vi "Idle_Password.vi"(2 "Called?":bool=TRUE) -> (0 "Correct?":bool, 1 "Access Level":i32)   [LabVIEW 2012]
uses:
  GlobalVariables_DIALMain.vi
  <vilib>/Utility/miscctls.llb/LVPointTypeDef.ctl
  <vilib>/Utility/miscctls.llb/LVRectTypeDef.ctl
panel:
  in  "Cancel":bool
  in  "Password":string
  in  "Set Password":bool
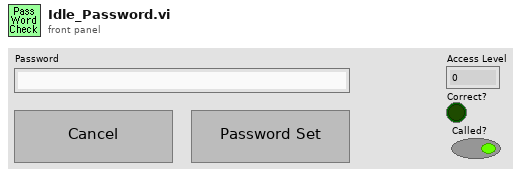
[diagram p1: front panel]
types:
  T1 = typedef "LVPointTypeDef.ctl" = cluster{"Horizontal":i16, "Vertical":i16}
  T2 = typedef "LVRectTypeDef.ctl" = cluster{"Left":i16, "Top":i16, "Right":i16, "Bottom":i16}
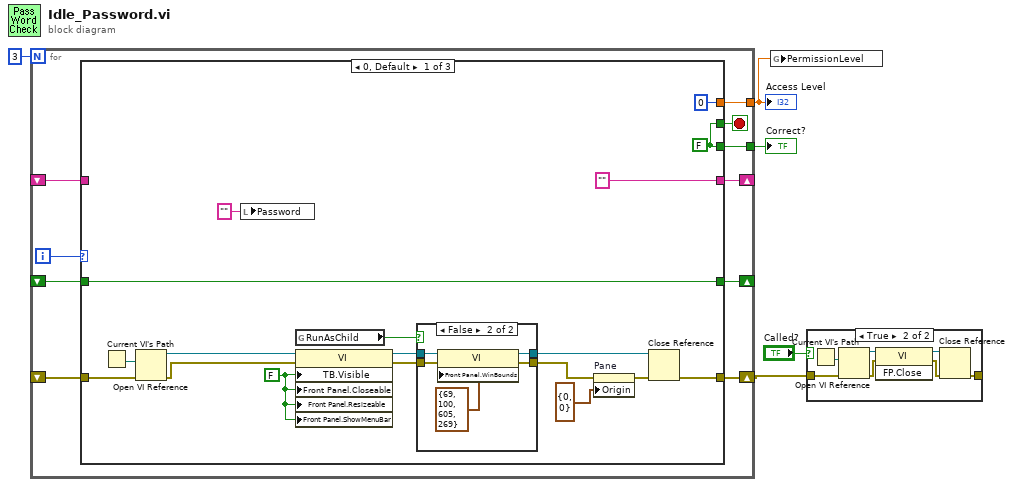
[diagram p0: block diagram]
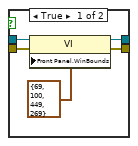
[diagram p3: hidden frame]
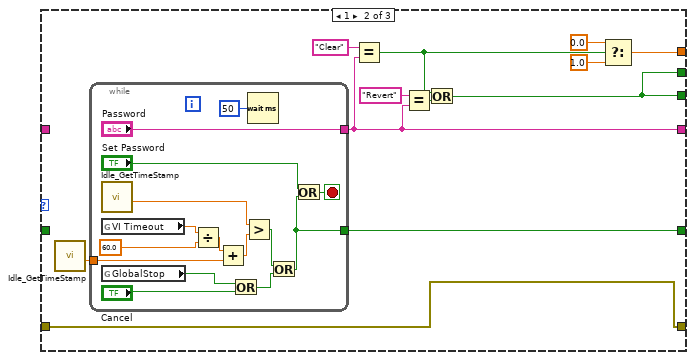
[diagram p4: hidden frame]
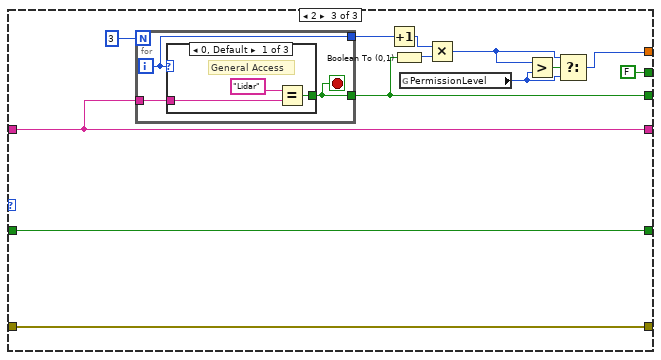
[diagram p5: hidden frame]
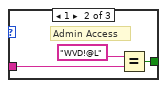
[diagram p6: hidden frame]
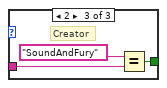
[diagram p7: hidden frame]
diagram:
  n1 = for {
    N: 3 -> [_]
    shift-right: [w14] -> _
    shift-left: _ -> [w11]
    shift-right: [w13] -> _
    shift-left: _ -> [w12]
    shift-right: [w9] -> w2
    shift-left: _ -> [w10]
    tunnel: [w8] -> w3
    tunnel: [w7] -> w4
    i -> [w15]
    stop <- w6 stop-if-true
    n2 = case shown="0, Default" w15 {
      tunnel: ["" ("Comment") w51 w82] -> w14
      tunnel: [w30 w54 w83] -> w13
      tunnel: w12 -> [w30 _ w83]
      tunnel: w11 -> [_ _ w82]
      tunnel: w10 -> [w29 w44 w71]
      tunnel: [w28 w44 w71] -> w9
      tunnel: [w25 w45 w78] -> w7
      tunnel: [0 w49 w74] -> w8
      tunnel: [w25 w45 FALSE] -> w6
      frame 0, Default {
        w25 = FALSE
        w33 = FALSE ("Tool Bar:Visible")
        n3 = Current VI's Path() -> (path=w32:path)
        n4 = Open VI Reference(vi path=w32, error in (no error)=w29) -> (vi reference=w17:refnum<vi>, error out=w16:errorcluster)  [unwired: 4 in]
        n5 = local write "Password"("" ("Password")) -> ()
        n6 = global read "GlobalVariables_DIALMain.vi" "RunAsChild"() -> (w18:bool)
        n7 = property class="VI"(reference=w17, error in=w16, "TB.Visible"=w33, "Front Panel.Closeable"=w33, "Front Panel.Resizeable"=w33, "Front Panel.ShowMenuBar"=w33) -> (reference out=w22:refnum<vi>, error out=w20:errorcluster)
        n8 = case shown="False" w18 {
          tunnel: w22 -> [w38 w43]
          tunnel: [w37 w42] -> w21
          tunnel: w20 -> [w36 w41]
          tunnel: [w35 w40] -> w19
          frame True {
            n9 = property class="VI"(reference=w38, error in=w36, "Front Panel.WinBounds"=T2 {"Left"=69, "Top"=100, "Right"=449, "Bottom"=269} ("Front Panel Window:Window Bounds 2")) -> (reference out=w37:refnum<vi>, error out=w35:errorcluster)
          }
          frame False {
            n10 = property class="VI"(reference=w43, error in=w41, "Front Panel.WinBounds"=T2 {"Left"=69, "Top"=100, "Right"=605, "Bottom"=269} ("Front Panel Window:Window Bounds 2")) -> (reference out=w42:refnum<vi>, error out=w40:errorcluster)
          }
        }
        n11 = property on="Pane" class="Pane"(error in=w19, "Origin"=T1 {"Horizontal"=0, "Vertical"=0}) -> (error out=w24:errorcluster)  [unwired: 1 in, 1 out]
        n12 = Close Reference(reference=w21, error in (no error)=w24) -> (error out=w28:errorcluster)
      }
      frame 1 {
        n13 = call "Idle_GetTimeStamp.vi"() -> ("Fractional Hours"=w55:dbl)  [unwired: 11 in]
        n14 = while {
          tunnel: ["Password"] -> w51
          tunnel: w55 -> [w62]
          tunnel: [w60] -> w54
          stop <- w63 stop-if-true
          n15 = call "Idle_GetTimeStamp.vi"() -> ("Fractional Hours"=w68:dbl)  [unwired: 11 in]
          n16 = global read "GlobalVariables_DIALMain.vi" "VI Timeout"() -> (w57:dbl)
          n17 = global read "GlobalVariables_DIALMain.vi" "GlobalStop"() -> (w56:bool)
          n18 = Divide(x=w57, y=60.0) -> (x/y=w65:dbl)
          n19 = Add(x=w65, y=w62) -> (x+y=w67:dbl)
          n20 = Or(x=w56, y="Cancel") -> (x .or. y?=w58:bool)
          n21 = Greater?(x=w68, y=w67) -> (0:w61:bool)
          n22 = Wait (ms)(milliseconds to wait=u32 50) -> ()  [unwired: 1 out]
          n23 = Or(x=w61, y=w58) -> (x .or. y?=w60:bool)
          n24 = Or(x="Set Password", y=w60) -> (x .or. y?=w63:bool)
        }
        n25 = Equal?(x="Clear" ("y"), y=w51) -> (x = y?=w46:bool)
        n26 = Equal?(x="Revert" ("y"), y=w51) -> (x = y?=w50:bool)
        n27 = Or(x=w46, y=w50) -> (x .or. y?=w45:bool)
        n28 = Select(t=0.0, s=w46, f=1.0) -> (s? t:f=w49:dbl)
      }
      frame 2 {
        n29 = for {
          N: 3 -> [_]
          tunnel: w82 -> [w86]
          tunnel: [w85] -> w78
          tunnel: [w84] -> w80
          i -> [w84]
          stop <- w85 stop-if-true
          n30 = case shown="0, Default" w84 {
            tunnel: w86 -> [w87 w90 w93]
            tunnel: [w88 w91 w94] -> w85
            frame 0, Default {
              # "General Access"
              n31 = Equal?(x="Lidar", y=w87) -> (x = y?=w88:bool)
            }
            frame 1 {
              # "Admin Access"
              n32 = Equal?(x="WVD!@L", y=w90) -> (x = y?=w91:bool)
            }
            frame 2 {
              # "Creator"
              n33 = Equal?(x="SoundAndFury", y=w93) -> (x = y?=w94:bool)
            }
          }
        }
        n34 = Increment(x=w80) -> (x+1=w79:i32)
        n35 = Boolean To (0,1)(Boolean=w78) -> (0, 1=w77:i16)
        n36 = global read "GlobalVariables_DIALMain.vi" "PermissionLevel"() -> (w72:i32)
        n37 = Multiply(x=w79, y=w77) -> (x*y=w75:i32)
        n38 = Greater?(x=w75, y=w72) -> (0:w76:bool)
        n39 = Select(t=w75, s=w76, f=w72) -> (s? t:f=w74:i32)
      }
    }
  }
  "Correct?" <- w4
  "Access Level" <- w3
  n40 = global write "GlobalVariables_DIALMain.vi" "PermissionLevel"(w3) -> ()
  n41 = case shown="True" "Called?" {
    tunnel: w2 -> [w96 w98]
    tunnel: [w96 w97] -> _
    frame False {
    }
    frame True {
      n42 = Current VI's Path() -> (path=w103:path)
      n43 = Open VI Reference(vi path=w103, error in (no error)=w98) -> (vi reference=w102:refnum<vi>, error out=w101:errorcluster)  [unwired: 4 in]
      n44 = invoke on="Invoke Node" class="VI" method="FP.Close"(reference=w102, error in=w101) -> (reference out=w99:refnum<vi>, error out=w100:errorcluster)  [unwired: 1 in, 1 out]
      n45 = Close Reference(reference=w99, error in (no error)=w100) -> (error out=w97:errorcluster)
    }
  }
